vi "TOL_EQ.vi"(8 "TOL VALUE":dbl, 11 "NOM VALUE":dbl) -> (0 "MIN":dbl, 3 "MAX":dbl)   [LabVIEW 2021]
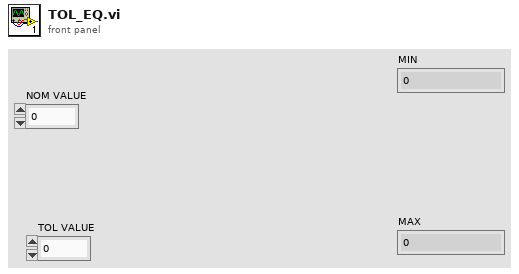
[diagram p1: front panel]
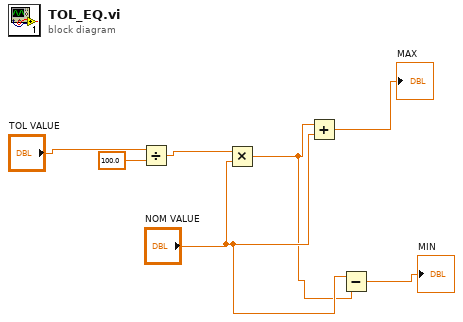
[diagram p0: block diagram]
diagram:
  n1 = Divide(x="TOL VALUE", y=100.0) -> (x/y=w5:dbl)
  n2 = Multiply(x=w5, y="NOM VALUE") -> (x*y=w1:dbl)
  n3 = Add(x=w1, y="NOM VALUE") -> (x+y=→"MAX":dbl)
  n4 = Subtract(x="NOM VALUE", y=w1) -> (x-y=→"MIN":dbl)
